vi "Add Task to Database.vi"(4 "Analog - Digital":bool, 5 "Total Acquisition Time":i32, 7 "DAQ Device Name":tag, 8 "error in":errorcluster, 9 "Digital Acquisition Parameters":T1 {"Execution Task Frequency" scale=1.0..100.0}, 10 "Analog Acquisition Parameters":T2={"sampling frequency Analog"=1000, "number of samples Analog"=1000, "Channels Analog"=[]} {"number of samples Analog" scale=0.0..2000.0; "sampling frequency Analog" scale=0.0..2000.0}) -> (0 "error out":errorcluster)   [LabVIEW 2020, in "Settings.lvlib"]
doc: "Request to add the specified configuration as a task to the Database.\n_____\nCreated using Delacor QMH Event Scripter 6.0.0.121."
uses:
  Settings.lvlib
  Shared/AnalogAcquisitionParameters__typedef.ctl
  Shared/DigitalAcquisitionParameters__typedef.ctl
  Add Task to Database Argument--cluster.ctl
  Shared/Configuration for Acquisitions.lvlib
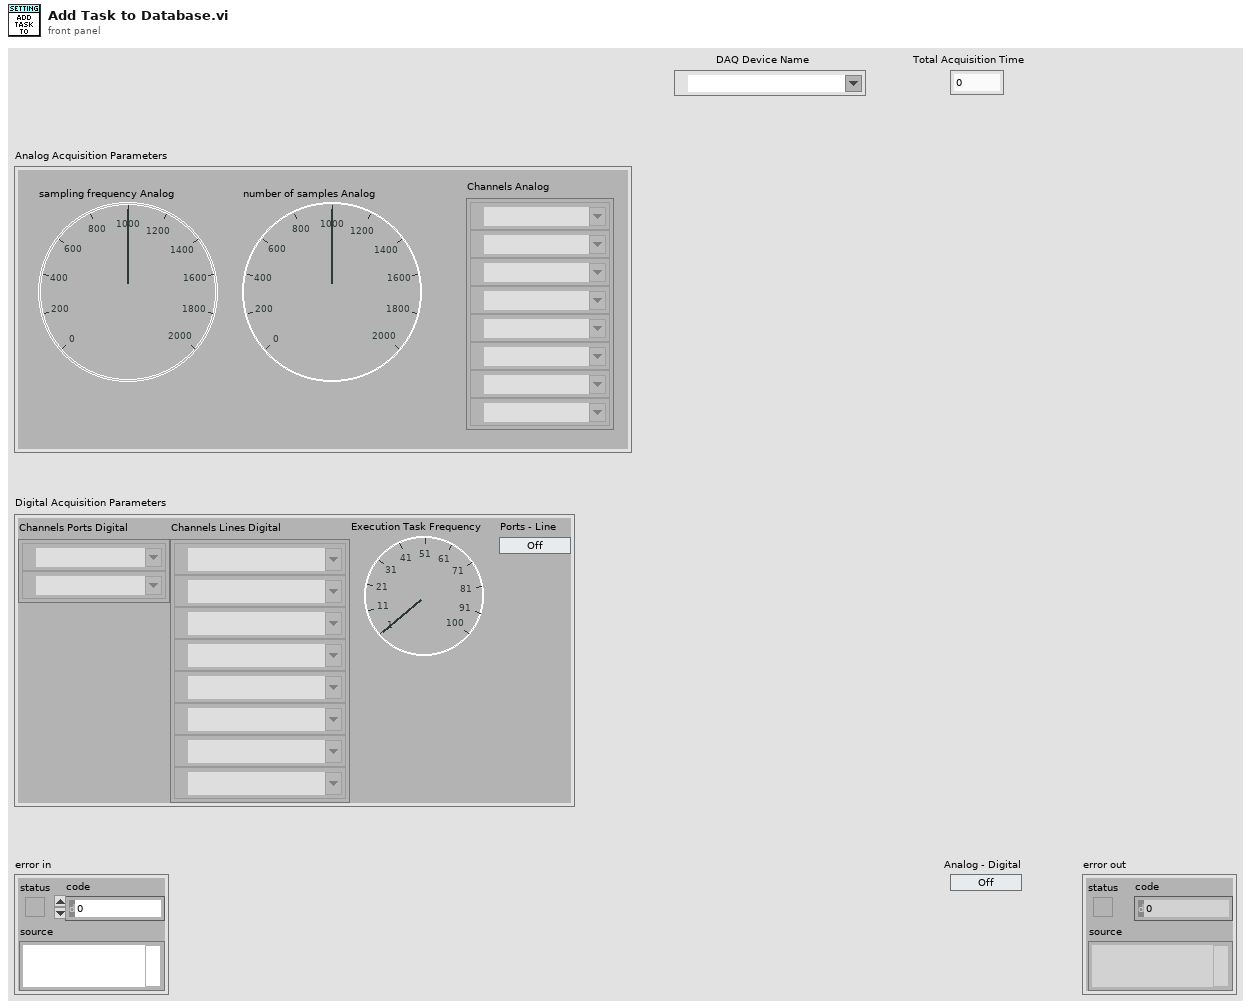
[diagram p1: front panel]
types:
  T1 = typedef "Configuration for Acquisitions.lvlib/DigitalAcquisitionParameters__typedef.ctl" = cluster{"Channels Ports Digital":tag[], "Channels Lines Digital":tag[], "Execution Task Frequency\n":u32, "Ports - Line":bool}
  T2 = typedef "Configuration for Acquisitions.lvlib/AnalogAcquisitionParameters__typedef.ctl" = cluster{"sampling frequency Analog":u32, "number of samples Analog":u32, "Channels Analog":tag[]}
  T3 = typedef "Settings.lvlib/Add Task to Database Argument--cluster.ctl" = cluster{"Analog Acquisition Parameters":T2, "Digital Acquisition Parameters":T1, "DAQ Device Name":tag, "Total Acquisition Time":i32, "Analog - Digital":bool}
  T4 = typedef "Settings.lvlib/Request Events--cluster.ctl" = cluster{"Stop Module":refnum<user-event>, "Show Panel":refnum<user-event>, "Hide Panel":refnum<user-event>, "Get Module Execution Status":refnum<user-event>, "Show Diagram":refnum<user-event>, "Add Task to Database":refnum<user-event>, "Erase All Tasks":refnum<user-event>}
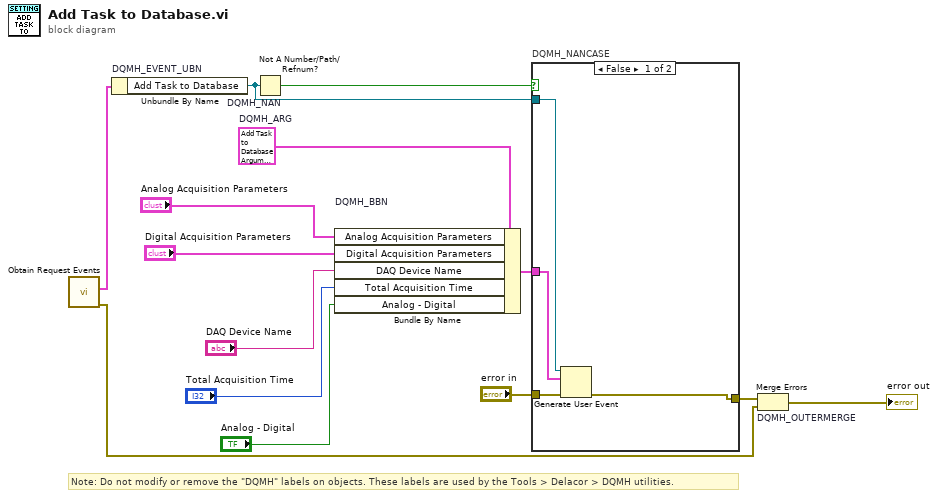
[diagram p0: block diagram]
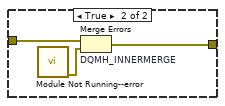
[diagram p2: hidden frame]
diagram:
  w8 = T3 {"Analog Acquisition Parameters"={"sampling frequency Analog"=1000, "number of samples Analog"=1000, "Channels Analog"=[]}, "Digital Acquisition Parameters"={"Channels Ports Digital"=[], "Channels Lines Digital"=[], "Execution Task Frequency\n"=0, "Ports - Line"=FALSE}, "DAQ Device Name"="", "Total Acquisition Time"=0, "Analog - Digital"=FALSE}  # DQMH_ARG
  # "Note: Do not modify or remove the \"DQMH\" labels on objects. These labels are used by the Tools > Delacor > DQMH utilities."
  n1 = call "Obtain Request Events.vi"() -> ("error out"=w2:errorcluster, "Settings Request Events"=w1:T4)  [unwired: 10 in]
  n2 = Unbundle By Name "DQMH_EVENT_UBN"(w1) -> ("Add Task to Database"=w10:refnum<user-event>)
  n3 = Not A Number/Path/Refnum? "DQMH_NAN"(number/path/refnum=w10) -> (NaN/Path/Refnum?=w11:bool)
  n4 = Bundle By Name "DQMH_BBN"(cluster=w8, "Analog Acquisition Parameters"="Analog Acquisition Parameters", "Digital Acquisition Parameters"="Digital Acquisition Parameters", "DAQ Device Name"="DAQ Device Name", "Total Acquisition Time"="Total Acquisition Time", "Analog - Digital"="Analog - Digital") -> (w12:T3)
  n5 = case "DQMH_NANCASE" shown="False" w11 {
    tunnel: "error in" -> [w18 w21]
    tunnel: [w17 w20] -> w9
    tunnel: w10 -> [w16 _]
    tunnel: w12 -> [w15 _]
    frame False {
      n6 = Generate User Event(user event=w16, event data cluster=w15, error in=w18) -> (error out=w17:errorcluster)  [unwired: 1 in, 1 out]
    }
    frame True {
      n7 = call "Module Not Running--error.vi"() -> ("error out"=w19:errorcluster)  [unwired: 11 in]
      n8 = Merge Errors "DQMH_INNERMERGE"(w21, w19) -> (w20:errorcluster)
    }
  }
  n9 = Merge Errors "DQMH_OUTERMERGE"(w9, w2) -> (→"error out":errorcluster)
